vi "Creating Cutom Probe.vi"() -> ()   [LabVIEW 2019]
panel:
  out "u32array":u32[](array[numeric])
  in  "stop":bool
  out "Value to Check":i32
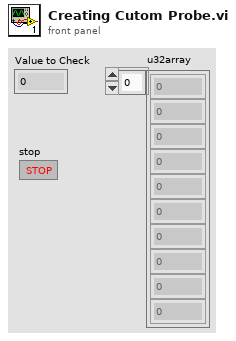
[diagram p1: front panel]
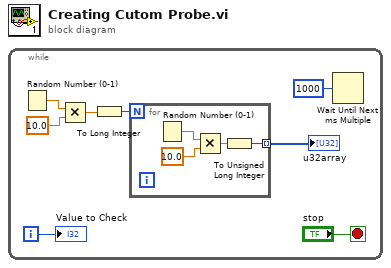
[diagram p0: block diagram]
diagram:
  n1 = while {
    i -> [w4]
    stop <- "stop" stop-if-true
    n2 = Random Number (0-1)() -> (number: 0 to 1=w5:dbl)
    n3 = Multiply(x=w5, y=10.0) -> (x*y=w7:dbl)
    n4 = To Long Integer(number=w7) -> (32bit integer=w8:i32)
    n5 = for {
      N: w8 -> [_]
      tunnel: [w9] -> w1 mode=indexing
      n6 = Random Number (0-1)() -> (number: 0 to 1=w11:dbl)
      n7 = Multiply(x=w11, y=10.0) -> (x*y=w10:dbl)
      n8 = To Unsigned Long Integer(number=w10) -> (unsigned 32bit integer=w9:u32)
    }
    "u32array" <- w1
    n9 = Wait Until Next ms Multiple(millisecond multiple=u32 1000) -> ()  [unwired: 1 out]
    "Value to Check" <- w4
  }
